vi "BGSub_Bella.vi"(8 "error in (no error)":errorcluster, 11 "raw Image In":T1) -> (0 "error out":errorcluster, 1 "Numeric":i32, 3 "Refnum out":T1, 4 "empty image":bool)   [LabVIEW 2013]
uses:
  IMAQ Image.ctl
  NI_Vision_Development_Module.lvlib
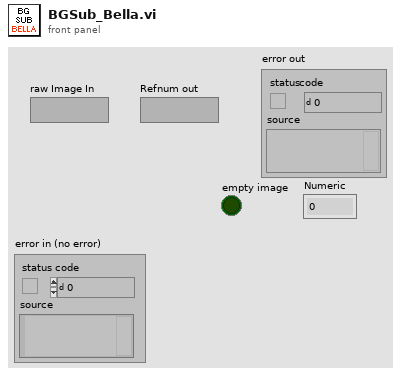
[diagram p1: front panel]
types:
  T1 = typedef "IMAQ Image.ctl" = refnum<image>
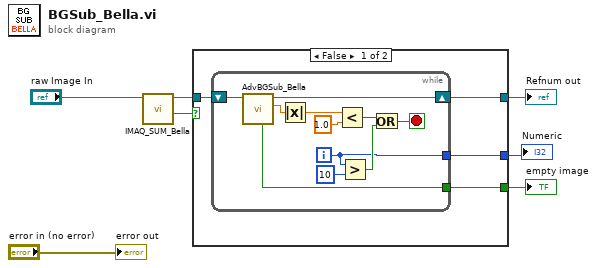
[diagram p0: block diagram]
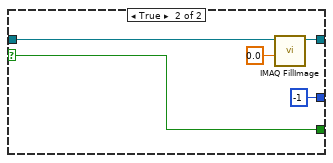
[diagram p2: hidden frame]
diagram:
  n1 = call "IMAQ_SUM_Bella.vi"("Image"="raw Image In") -> ("empty Image"=w1:bool, "Image out"=w5:T1)  [unwired: 8 in, 1 out]
  n2 = case shown="False" w1 {
    selector: w1 -> [_ w23]
    tunnel: [w11 w25] -> w4
    tunnel: w5 -> [w10 w27]
    tunnel: [w9 w23] -> w7
    tunnel: [w8 -1] -> w2
    frame False {
      n3 = while {
        shift-right: [w15] -> w11
        shift-left: w10 -> [w16]
        tunnel: [w13] -> w9
        tunnel: [w12] -> w8
        i -> [w12]
        stop <- w22 stop-if-true
        n4 = call "AdvBGSub_Bella.vi"("Refnum in"=w16) -> ("-x"=w14:sgl, "Refnum out"=w15:T1, "empty image"=w13:bool)  [unwired: 7 in, 1 out]
        n5 = Absolute Value(x=w14) -> (abs(x)=w17:sgl)
        n6 = Less?(x=w17, y=sgl 1.0) -> (x < y?=w20:bool)
        n7 = Greater?(x=w12, y=10) -> (0:w18:bool)
        n8 = Or(x=w20, y=w18) -> (x .or. y?=w22:bool)
      }
    }
    frame True {
      n9 = call "IMAQ FillImage"("Pixel Value (U8, U16, I16, Float)"=sgl 0.0, "Image"=w27) -> ("Image Out"=w25:T1)  [unwired: 8 in, 1 out]
    }
  }
  "Refnum out" <- w4
  "empty image" <- w7
  "Numeric" <- w2
  "error out" <- "error in (no error)"
